vi "查询上序合格.vi"(8 "error in (no error)":errorcluster, 11 "产品ID":string="123456") -> (0 "error out":errorcluster, 1 "本序已做":bool, 2 "上序合格":bool)   [LabVIEW 2013]
uses:
  <vilib>/Utility/error.llb/whitespace.ctl
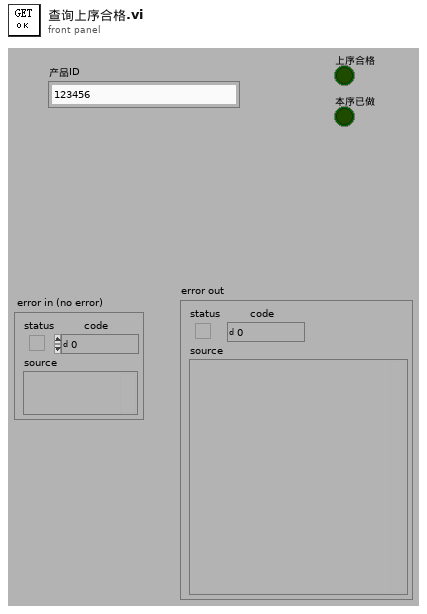
[diagram p1: front panel]
types:
  T1 = typedef "whitespace.ctl" = u16
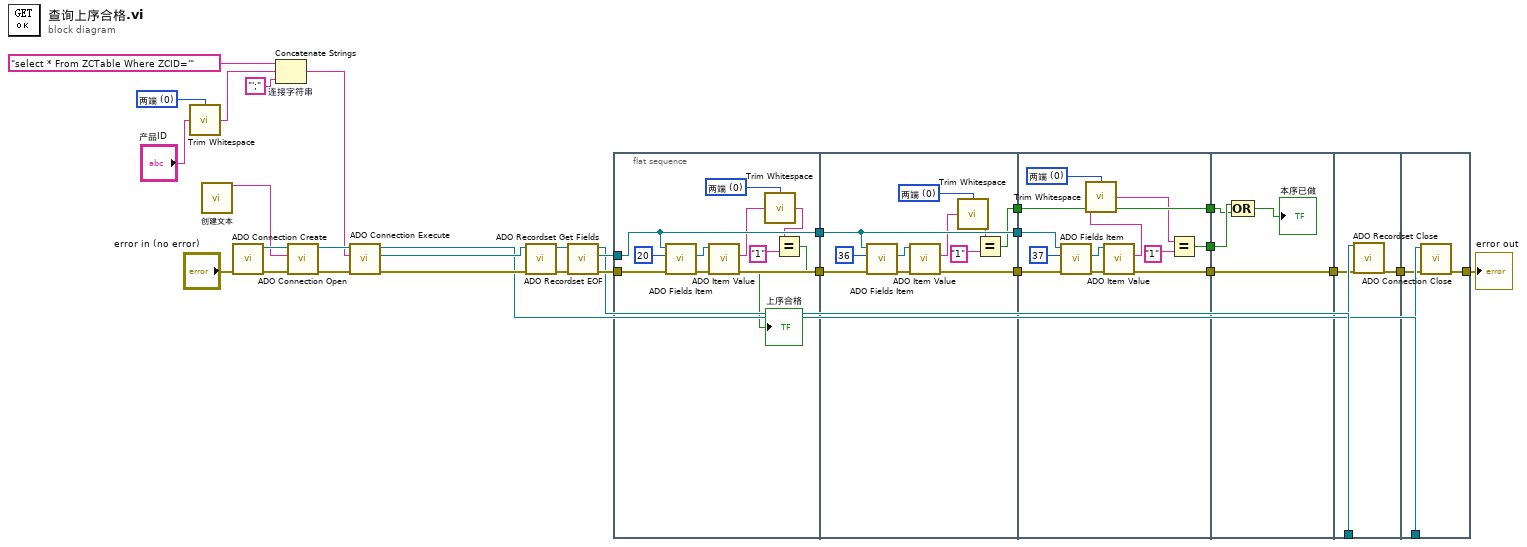
[diagram p0: block diagram]
diagram:
  w21 = T1 0 items=["两端", "字符串首端", "字符串末端"] ("location (both)")
  n1 = call <vilib>:"Trim Whitespace.vi"("string"="产品ID", "location (both)"=w21) -> ("trimmed string"=w22:string)
  n2 = call "创建文本"() -> ("Result"=w1:string)  [unwired: 14 in, 1 out]
  n3 = call "ADO Connection Create.vi"("error in (no error)"="error in (no error)") -> ("error out"=w30:errorcluster, "ADODB._Connection Out"=w31:refnum<k7>)  [unwired: 9 out]
  n4 = Concatenate Strings "连接字符串"("select * From ZCTable Where ZCID='" ("字符串 2"), w22, "';" ("字符串 2")) -> (w20:string)
  n5 = call "ADO Connection Open.vi"("error in (no error)"=w30, "ConnectionString"=w1, "ADODB._Connection In"=w31) -> ("error out"=w29:errorcluster, "ADODB._Connection Out"=w28:refnum<k7>)  [unwired: 7 out]
  n6 = call "ADO Connection Execute.vi"("error in (no error)"=w29, "CommandText"=w20, "ADODB._Connection In"=w28) -> ("error out"=w26:errorcluster, "RecordSet"=w27:refnum<k7>, "ADODB._Connection Out"=w12:refnum<k7>)  [unwired: 6 out]
  n7 = call "ADO Recordset EOF.vi"("error in (no error)"=w26, "ADODB._Recordset In"=w27) -> ("error out"=w17:errorcluster, "ADODB._Recordset Out"=w18:refnum<k7>)  [unwired: 8 out]
  n8 = call "ADO Recordset Get Fields.vi"("error in (no error)"=w17, "ADODB._Recordset In"=w18) -> ("error out"=w15:errorcluster, "Fields Out"=w16:refnum<k7>, "ADODB._Recordset Out"=w13:refnum<k7>)  [unwired: 7 out]
  n9 = flat-sequence {
    tunnel: w16 -> [w37]
    tunnel: w15 -> [w38]
    tunnel: [w42] -> w9
    tunnel: [w37] -> w8
    tunnel: w9 -> [w50]
    tunnel: w8 -> [w47]
    tunnel: [w49] -> w6
    tunnel: [w47] -> w5
    tunnel: [w46] -> w3
    tunnel: [w61] -> w7
    tunnel: w6 -> [w62]
    tunnel: w5 -> [w59]
    tunnel: [w58] -> w4
    tunnel: w3 -> [w57]
    tunnel: [w57] -> w2
    tunnel: w7 -> [w69]
    tunnel: [w69] -> w14
    tunnel: w4 -> [w68]
    tunnel: w2 -> [w67]
    tunnel: w14 -> [w71]
    tunnel: w13 -> [w72]
    tunnel: [w70] -> w11
    tunnel: w12 -> [w75]
    tunnel: w11 -> [w74]
    tunnel: [w73] -> w10
    frame #0 {
      w35 = T1 0 items=["两端", "字符串首端", "字符串末端"] ("location (both)")
      n10 = call "ADO Fields Item.vi"("error in (no error)"=w38, "Index"=20, "Fields In"=w37) -> ("error out"=w40:errorcluster, "Item Out"=w39:refnum<k7>)  [unwired: 7 out]
      n11 = call "ADO Item Value.vi"("error in (no error)"=w40, "Item In"=w39) -> ("error out"=w42:errorcluster, "Value"=w34:string)  [unwired: 8 out]
      n12 = call <vilib>:"Trim Whitespace.vi"("string"=w34, "location (both)"=w35) -> ("trimmed string"=w33:string)
      n13 = Equal?(x=w33, y="1") -> (x = y?=→"上序合格":bool)
    }
    frame #1 {
      w45 = T1 0 items=["两端", "字符串首端", "字符串末端"] ("location (both)")
      n14 = call "ADO Fields Item.vi"("error in (no error)"=w50, "Index"=36, "Fields In"=w47) -> ("error out"=w52:errorcluster, "Item Out"=w51:refnum<k7>)  [unwired: 7 out]
      n15 = call "ADO Item Value.vi"("error in (no error)"=w52, "Item In"=w51) -> ("error out"=w49:errorcluster, "Value"=w44:string)  [unwired: 8 out]
      n16 = call <vilib>:"Trim Whitespace.vi"("string"=w44, "location (both)"=w45) -> ("trimmed string"=w43:string)
      n17 = Equal?(x=w43, y="1") -> (x = y?=w46:bool)
    }
    frame #2 {
      w56 = T1 0 items=["两端", "字符串首端", "字符串末端"] ("location (both)")
      n18 = call "ADO Fields Item.vi"("error in (no error)"=w62, "Index"=37, "Fields In"=w59) -> ("error out"=w64:errorcluster, "Item Out"=w63:refnum<k7>)  [unwired: 7 out]
      n19 = call "ADO Item Value.vi"("error in (no error)"=w64, "Item In"=w63) -> ("error out"=w61:errorcluster, "Value"=w55:string)  [unwired: 8 out]
      n20 = call <vilib>:"Trim Whitespace.vi"("string"=w55, "location (both)"=w56) -> ("trimmed string"=w54:string)
      n21 = Equal?(x=w54, y="1") -> (x = y?=w58:bool)
    }
    frame #3 {
      n22 = Compound Arithmetic op=OR(w68, w67) -> (→"本序已做":bool)
    }
    frame #4 {
      n23 = call "ADO Recordset Close.vi"("ADODB._Recordset In"=w72, "error in (no error)"=w71) -> ("error out"=w70:errorcluster)  [unwired: 17 out]
    }
    frame #5 {
      n24 = call "ADO Connection Close.vi"("error in (no error)"=w74, "ADODB._Connection In"=w75) -> ("error out"=w73:errorcluster)  [unwired: 9 out]
    }
  }
  "error out" <- w10
